vi "Z900_navX_Util_DecodeProtocol_SignedRatio.vi"(1 "Little Endian":u8[](array[numeric])) -> (0 "Signed Ratio":dbl[](array[numeric]))   [LabVIEW 2015, in "navX Library v2.lvlib"]
uses:
  navX Library v2.lvlib
  Z900_navX_Util_LittleEndian_to_BigEndian.vi
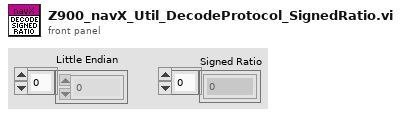
[diagram p1: front panel]
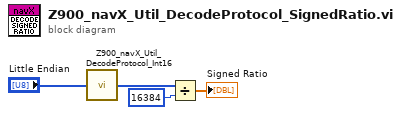
[diagram p0: block diagram]
diagram:
  n1 = call "Z900_navX_Util_DecodeProtocol_Int16.vi"("Little Endian"="Little Endian") -> ("Int16"=w3:i16[])
  n2 = Divide(x=w3, y=u16 16384) -> (x/y=→"Signed Ratio":dbl[])
